vi "solar_type Get Type.vi"(0 "Variant":variant) -> (4 "Type":T1, 5 "Name":string, 6 "Enum Names":string[](array[string]))   [LabVIEW 2018]
doc: "This VI returns the data type of the variant. Not all data types are supported. Array of clusters are not supported."
uses:
  solar_type Item Type.ctl
  <vilib>/Utility/Data Type/NI_Data Type.lvlib
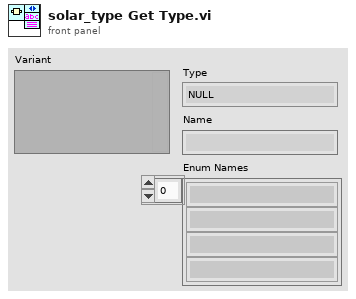
[diagram p1: front panel]
types:
  T1 = typedef "solar_type Item Type.ctl" = enum16{"NULL", "UNKNOWN", "CLUSTER", "I8", "I16", "I32", "I64", "U8", "U16", "U32", "U64", "U8_ENUM", "U16_ENUM", "U32_ENUM", "SGL", "DBL", "BOOLEAN", "STRING", "PATH", "VISA", "TAG", "TIME", "I8_1D", "I16_1D", "I32_1D", "I64_1D", "U8_1D", "U16_1D", "U32_1D", "U64_1D", "U8_ENUM_1D", "U16_ENUM_1D", "U32_ENUM_1D", "SGL_1D", "DBL_1D", "BOOLEAN_1D", "STRING_1D", "PATH_1D", "VISA_1D", "TAG_1D", "TIME_1D", "I8_2D", "I16_2D", "I32_2D", "I64_2D", "U8_2D", "U16_2D", "U32_2D", "U64_2D", "U8_ENUM_2D", "U16_ENUM_2D", "U32_ENUM_2D", "SGL_2D", "DBL_2D", "BOOLEAN_2D", "STRING_2D", "PATH_2D", "VISA_2D", "TAG_2D", "TIME_2D"}
  T2 = typedef "NI_Data Type.lvlib/Data Type.ctl" = enum8{"Invalid Type", "Void", "I8", "I16", "I32", "I64", "U8", "U16", "U32", "U64", "Single Float", "Double Float", "Extended Float", "Single Complex", "Double Complex", "Extended Complex", "Enum U8", "Enum U16", "Enum U32", "Enum U64", "Single Float With Unit", "Double Float With Unit", "Extended Float With Unit", "Single Complex with Unit", "Double Complex with Unit", "Extended Complex with Unit", "Boolean", "String", "Path", "Picture", "Tag", "Array", "Cluster", "Variant", "LV Variant", "Waveform", "Timestamp", "Digital Waveform", "Digital Data", "ExpressData", "Refnum", "External Data", "VI", "Poly VI", "LabVIEW Class Instance", "Fixed Point", "Set Collection", "Map Collection"}
  T3 = typedef "NI_Data Type.lvlib/Refnum Type.ctl" = enum16{"NotARefnum", "UnknownRefnum", "Generic", "Datalog", "ByteStream", "Device", "Occurence", "TCPNetConnection", "Auto", "Menu", "Imaq", "Hardware", "DataSocket", "Visa", "IVI", "UDPNetConnection", "Notifier", "Queue", "Irda", "EventReg", "DotNet", "UserEvent", "Callback", "UNUSED_EMPTY_POSITION", "BlueToothNetConnection", "LVObjApp", "LVObjVI", "LVObjUnknown", "GenericClass", "UserDefinedRefnumTag", "DataValue", "RT FIFO", "TDMS File", "PythonSessionRefnum"}
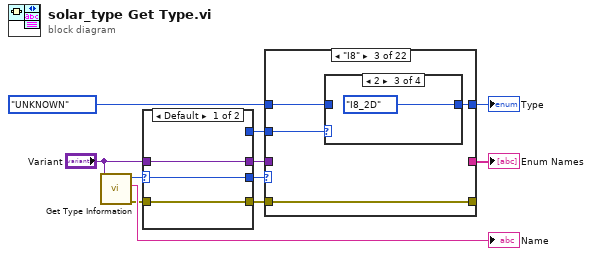
[diagram p0: block diagram]
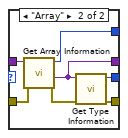
[diagram p2: hidden frame]
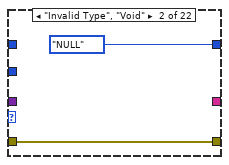
[diagram p4: hidden frame]
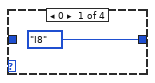
[diagram p5: hidden frame]
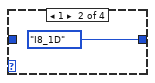
[diagram p6: hidden frame]
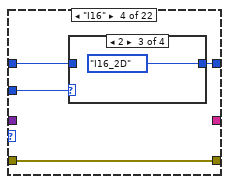
[diagram p8: hidden frame]
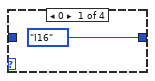
[diagram p9: hidden frame]
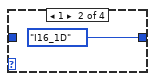
[diagram p10: hidden frame]
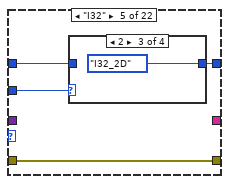
[diagram p12: hidden frame]
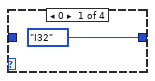
[diagram p13: hidden frame]
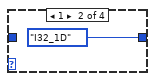
[diagram p14: hidden frame]
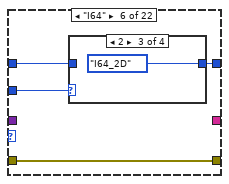
[diagram p16: hidden frame]
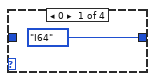
[diagram p17: hidden frame]
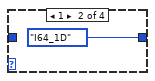
[diagram p18: hidden frame]
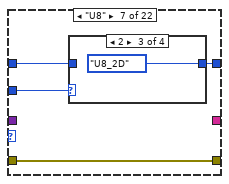
[diagram p20: hidden frame]
diagram:
  n1 = call <vilib>:"Get Type Information.vi"("variant"="Variant") -> ("error out"=w2:errorcluster, "name"=→"Name":string, "type"=w5:T2)  [unwired: 6 in, 2 out]
  n2 = case shown="Default" w5 {
    selector: w5 -> [w14 _]
    tunnel: "Variant" -> [w13 w21]
    tunnel: [_ w20] -> w9
    tunnel: [w14 w19] -> w8
    tunnel: [w13 w18] -> w7
    tunnel: w2 -> [w12 w17]
    tunnel: [w12 w15] -> w1
    frame Default {
    }
    frame "Array" {
      n3 = call <vilib>:"Get Array Information.vi"("error in (no error)"=w17, "variant"=w21) -> ("error out"=w16:errorcluster, "array element data type"=w18:variant, "number of dimensions"=w20:i32)  [unwired: 6 in, 1 out]
      n4 = call <vilib>:"Get Type Information.vi"("error in (no error)"=w16, "variant"=w18) -> ("error out"=w15:errorcluster, "type"=w19:T2)  [unwired: 5 in, 3 out]
    }
  }
  n5 = case shown="\"I8\"" w8 {
    tunnel: [w23 solar_type_Item_Type."NULL" ("Type 2") w29 w37 w45 w53 w61 w69 w77 w85 w93 w101 w112 w123 w134 w143 w151 w159 w167 w175 w185 w197] -> w11
    tunnel: w9 -> [_ _ w28 w36 w44 w52 w60 w68 w76 w84 w92 w100 w111 w122 w133 w142 w150 w158 w166 w174 w184 w196]
    tunnel: w7 -> [_ _ _ _ _ _ _ _ _ _ _ _ w109 w120 w131 _ _ _ _ _ w182 _]
    tunnel: solar_type_Item_Type."UNKNOWN" ("Type 2") -> [w23 _ w27 w35 w43 w51 w59 w67 w75 w83 w91 w99 w110 w121 w132 w141 w149 w157 w165 w173 w183 w195]
    tunnel: [_ _ _ _ _ _ _ _ _ _ _ _ w108 w119 w130 string[] ["false", "true"] ("Enum Names") _ _ _ _ _ _] -> w3
    tunnel: w1 -> [w22 w24 w26 w34 w42 w50 w58 w66 w74 w82 w90 w98 w107 w118 w129 w140 w148 w156 w164 w172 w180 w194]
    tunnel: [w22 w24 w26 w34 w42 w50 w58 w66 w74 w82 w90 w98 w106 w117 w128 w140 w148 w156 w164 w172 w180 w194] -> _
    frame Default {
    }
    frame "Invalid Type", "Void" {
    }
    frame "I8" {
      n6 = case shown="2" w28 {
        tunnel: [solar_type_Item_Type."I8" ("Type 2") solar_type_Item_Type."I8_1D" ("Type 2") solar_type_Item_Type."I8_2D" ("Type 2") w33] -> w29
        tunnel: w27 -> [_ _ _ w33]
        frame 0 {
        }
        frame 1 {
        }
        frame 2 {
        }
        frame Default {
        }
      }
    }
    frame "I16" {
      n7 = case shown="2" w36 {
        tunnel: [solar_type_Item_Type."I16" ("Type 2") solar_type_Item_Type."I16_1D" ("Type 2") solar_type_Item_Type."I16_2D" ("Type 2") w41] -> w37
        tunnel: w35 -> [_ _ _ w41]
        frame 0 {
        }
        frame 1 {
        }
        frame 2 {
        }
        frame Default {
        }
      }
    }
    frame "I32" {
      n8 = case shown="2" w44 {
        tunnel: [solar_type_Item_Type."I32" ("Type 2") solar_type_Item_Type."I32_1D" ("Type 2") solar_type_Item_Type."I32_2D" ("Type 2") w49] -> w45
        tunnel: w43 -> [_ _ _ w49]
        frame 0 {
        }
        frame 1 {
        }
        frame 2 {
        }
        frame Default {
        }
      }
    }
    frame "I64" {
      n9 = case shown="2" w52 {
        tunnel: [solar_type_Item_Type."I64" ("Type 2") solar_type_Item_Type."I64_1D" ("Type 2") solar_type_Item_Type."I64_2D" ("Type 2") w57] -> w53
        tunnel: w51 -> [_ _ _ w57]
        frame 0 {
        }
        frame 1 {
        }
        frame 2 {
        }
        frame Default {
        }
      }
    }
    frame "U8" {
      n10 = case shown="2" w60 {
        tunnel: [solar_type_Item_Type."U8" ("Type 2") solar_type_Item_Type."U8_1D" ("Type 2") solar_type_Item_Type."U8_2D" ("Type 2") w65] -> w61
        tunnel: w59 -> [_ _ _ w65]
        frame 0 {
        }
        frame 1 {
        }
        frame 2 {
        }
        frame Default {
        }
      }
    }
    frame "U16" {
      n11 = case shown="2" w68 {
        tunnel: [solar_type_Item_Type."U16" ("Type 2") solar_type_Item_Type."U16_1D" ("Type 2") solar_type_Item_Type."U16_2D" ("Type 2") w73] -> w69
        tunnel: w67 -> [_ _ _ w73]
        frame 0 {
        }
        frame 1 {
        }
        frame 2 {
        }
        frame Default {
        }
      }
    }
    frame "U32" {
      n12 = case shown="2" w76 {
        tunnel: [solar_type_Item_Type."U32" ("Type 2") solar_type_Item_Type."U32_1D" ("Type 2") solar_type_Item_Type."U32_2D" ("Type 2") w81] -> w77
        tunnel: w75 -> [_ _ _ w81]
        frame 0 {
        }
        frame 1 {
        }
        frame 2 {
        }
        frame Default {
        }
      }
    }
    frame "U64" {
      n13 = case shown="2" w84 {
        tunnel: [solar_type_Item_Type."U64" ("Type 2") solar_type_Item_Type."U64_1D" ("Type 2") solar_type_Item_Type."U64_2D" ("Type 2") w89] -> w85
        tunnel: w83 -> [_ _ _ w89]
        frame 0 {
        }
        frame 1 {
        }
        frame 2 {
        }
        frame Default {
        }
      }
    }
    frame "Single Float", "Single Float With Unit" {
      n14 = case shown="2" w92 {
        tunnel: [solar_type_Item_Type."SGL" ("Type 2") solar_type_Item_Type."SGL_1D" ("Type 2") solar_type_Item_Type."SGL_2D" ("Type 2") w97] -> w93
        tunnel: w91 -> [_ _ _ w97]
        frame 0 {
        }
        frame 1 {
        }
        frame 2 {
        }
        frame Default {
        }
      }
    }
    frame "Double Float", "Double Float With Unit" {
      n15 = case shown="2" w100 {
        tunnel: [solar_type_Item_Type."DBL" ("Type 2") solar_type_Item_Type."DBL_1D" ("Type 2") solar_type_Item_Type."DBL_2D" ("Type 2") w105] -> w101
        tunnel: w99 -> [_ _ _ w105]
        frame 0 {
        }
        frame 1 {
        }
        frame 2 {
        }
        frame Default {
        }
      }
    }
    frame "Enum U8" {
      n16 = call <vilib>:"Get Numeric Information.vi"("error in (no error)"=w107, "variant"=w109) -> ("error out"=w106:errorcluster, "enum names"=w108:string[])  [unwired: 6 in, 2 out]
      n17 = case shown="Default" w111 {
        tunnel: [solar_type_Item_Type."U8_ENUM" ("Type 2") solar_type_Item_Type."U8_ENUM_1D" ("Type 2") solar_type_Item_Type."U8_ENUM_2D" ("Type 2") w116] -> w112
        tunnel: w110 -> [_ _ _ w116]
        frame 0 {
        }
        frame 1 {
        }
        frame 2 {
        }
        frame Default {
        }
      }
    }
    frame "Enum U16" {
      n18 = call <vilib>:"Get Numeric Information.vi"("error in (no error)"=w118, "variant"=w120) -> ("error out"=w117:errorcluster, "enum names"=w119:string[])  [unwired: 6 in, 2 out]
      n19 = case shown="2" w122 {
        tunnel: [solar_type_Item_Type."U16_ENUM" ("Type 2") solar_type_Item_Type."U16_ENUM_1D" ("Type 2") solar_type_Item_Type."U16_ENUM_2D" ("Type 2") w127] -> w123
        tunnel: w121 -> [_ _ _ w127]
        frame 0 {
        }
        frame 1 {
        }
        frame 2 {
        }
        frame Default {
        }
      }
    }
    frame "Enum U32" {
      n20 = call <vilib>:"Get Numeric Information.vi"("error in (no error)"=w129, "variant"=w131) -> ("error out"=w128:errorcluster, "enum names"=w130:string[])  [unwired: 6 in, 2 out]
      n21 = case shown="2" w133 {
        tunnel: [solar_type_Item_Type."U32_ENUM" ("Type 2") solar_type_Item_Type."U32_ENUM_1D" ("Type 2") solar_type_Item_Type."U32_ENUM_2D" ("Type 2") w138] -> w134
        tunnel: w132 -> [_ _ _ w138]
        frame 0 {
        }
        frame 1 {
        }
        frame 2 {
        }
        frame Default {
        }
      }
    }
    frame "Boolean" {
      n22 = case shown="2" w142 {
        tunnel: [solar_type_Item_Type."BOOLEAN" ("Type 2") solar_type_Item_Type."BOOLEAN_1D" ("Type 2") solar_type_Item_Type."BOOLEAN_2D" ("Type 2") w147] -> w143
        tunnel: w141 -> [_ _ _ w147]
        frame 0 {
        }
        frame 1 {
        }
        frame 2 {
        }
        frame Default {
        }
      }
    }
    frame "String" {
      n23 = case shown="2" w150 {
        tunnel: [solar_type_Item_Type."STRING" ("Type 2") solar_type_Item_Type."STRING_1D" ("Type 2") solar_type_Item_Type."STRING_2D" ("Type 2") w155] -> w151
        tunnel: w149 -> [_ _ _ w155]
        frame 0 {
        }
        frame 1 {
        }
        frame 2 {
        }
        frame Default {
        }
      }
    }
    frame "Path" {
      n24 = case shown="2" w158 {
        tunnel: [solar_type_Item_Type."PATH" ("Type 2") solar_type_Item_Type."PATH_1D" ("Type 2") solar_type_Item_Type."PATH_2D" ("Type 2") w163] -> w159
        tunnel: w157 -> [_ _ _ w163]
        frame 0 {
        }
        frame 1 {
        }
        frame 2 {
        }
        frame Default {
        }
      }
    }
    frame "Tag" {
      n25 = case shown="2" w166 {
        tunnel: [solar_type_Item_Type."TAG" ("Type 2") solar_type_Item_Type."TAG_1D" ("Type 2") solar_type_Item_Type."TAG_2D" ("Type 2") w171] -> w167
        tunnel: w165 -> [_ _ _ w171]
        frame 0 {
        }
        frame 1 {
        }
        frame 2 {
        }
        frame Default {
        }
      }
    }
    frame "Timestamp" {
      n26 = case shown="2" w174 {
        tunnel: [solar_type_Item_Type."TIME" ("Type 2") solar_type_Item_Type."TIME_1D" ("Type 2") solar_type_Item_Type."TIME_2D" ("Type 2") w179] -> w175
        tunnel: w173 -> [_ _ _ w179]
        frame 0 {
        }
        frame 1 {
        }
        frame 2 {
        }
        frame Default {
        }
      }
    }
    frame "Refnum" {
      n27 = call <vilib>:"Get Refnum Information.vi"("variant"=w182) -> ("reference type"=w181:T3)  [unwired: 7 in, 3 out]
      n28 = case shown="\"Visa\"" w181 {
        tunnel: [w186 w189] -> w185
        tunnel: w184 -> [_ w188]
        tunnel: w183 -> [w186 w187]
        frame Default {
        }
        frame "Visa" {
          n29 = case shown="2" w188 {
            tunnel: [solar_type_Item_Type."VISA" ("Type 2") solar_type_Item_Type."VISA_1D" ("Type 2") solar_type_Item_Type."VISA_2D" ("Type 2") w193] -> w189
            tunnel: w187 -> [_ _ _ w193]
            frame 0 {
            }
            frame 1 {
            }
            frame 2 {
            }
            frame Default {
            }
          }
        }
      }
    }
    frame "Cluster" {
      n30 = case shown="0" w196 {
        tunnel: [solar_type_Item_Type."CLUSTER" ("Type 2") w199] -> w197
        tunnel: w195 -> [_ w199]
        frame 0 {
        }
        frame Default {
        }
      }
    }
  }
  "Type" <- w11
  "Enum Names" <- w3
